vi "demo_constants.vi"   [LabVIEW 2021]
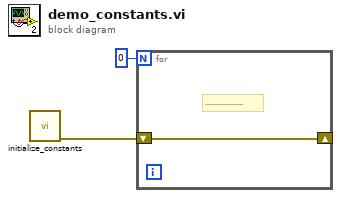
[diagram p0: block diagram]
diagram:
  n1 = call "initialize_constants.vi"() -> ("error out"=w2:errorcluster)  [unwired: 11 in]
  n2 = for {
    N: 0 -> [_]
    shift-right: [w3] -> _
    shift-left: w2 -> [w3]
    # "..................."
  }
